vi "FTW-Endpoint-CreateRequester.vi"(0 "FTW Endpoint":refnum<class "FTW-Endpoint-TCP.lvclass">, 5 "Endpoint Address":string, 11 "error in":errorcluster) -> (4 "FTW Endpoint out":refnum<class "FTW-Endpoint-TCP.lvclass">, 15 "error out":errorcluster)   [LabVIEW 2013, in "FTW-Endpoint-TCP.lvclass"]
uses:
  FTW-Endpoint-TCP.lvclass
  Endpoint/FTW-Endpoint.lvclass
  FTW-Endpoint-TCP.lvclass/FTW-Endpoint-TCP.ctl
panel:
  # "Inputs"
  # "Outputs"
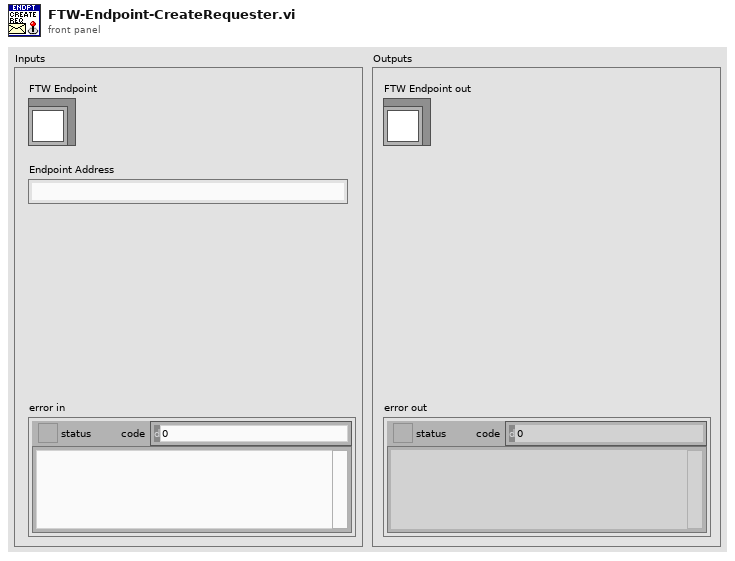
[diagram p1: front panel]
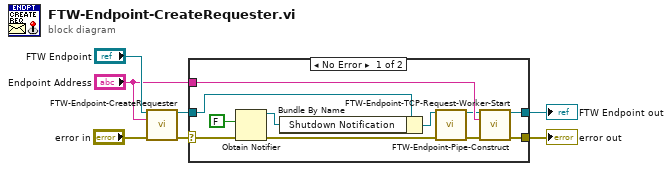
[diagram p0: block diagram]
diagram:
  n1 = call-parent "FTW-Endpoint-CreateRequester.vi"("FTW Endpoint"="FTW Endpoint", "Endpoint Address"="Endpoint Address", "error in"="error in") -> ("FTW Endpoint out"=w6:refnum<class "FTW-Endpoint-TCP.lvclass">, "error out"=w4:errorcluster)  [unwired: 11 in]
  n2 = case shown="No Error" w4 {
    selector: w4 -> [w12 w19]
    tunnel: w6 -> [w11 w20]
    tunnel: [w13 w20] -> w3
    tunnel: [w15 w19] -> w2
    tunnel: "Endpoint Address" -> [w16 _]
    frame No Error {
      n3 = Obtain Notifier(notification data type=FALSE, error in (no error)=w12) -> (notifier out=w14:refnum<notifier>, error out=w17:errorcluster)  [unwired: 2 in, 1 out]
      n4 = Bundle By Name(cluster=w11, "Shutdown Notification"=w14) -> (w9:refnum<class "FTW-Endpoint-TCP.lvclass">)
      n5 = call-dynamic "FTW-Endpoint-Pipe-Construct.vi"("FTW Endpoint"=w9, "error in"=w17) -> ("FTW Endpoint out"=w8:refnum<class "FTW-Endpoint-TCP.lvclass">, "error out"=w10:errorcluster)  [unwired: 11 in, 1 out]
      n6 = call-dynamic "FTW-Endpoint-TCP-Request-Worker-Start.vi"("FTW-Endpoint-TCP In"=w8, "Endpoint Address"=w16, "error in"=w10) -> ("FTW-Endpoint-TCP Out"=w13:refnum<class "FTW-Endpoint-TCP.lvclass">, "error out"=w15:errorcluster)  [unwired: 11 in]
    }
    frame Error {
    }
  }
  "error out" <- w2
  "FTW Endpoint out" <- w3
